vi "GetControlRef.vi"(0 "reference in":refnum<class "MLA.lvclass">, 1 "Control Label":string, 2 "Control Class":string, 5 "error in (no error)":errorcluster) -> (14 "reference out":refnum<class "MLA.lvclass">, 15 "Control":refnum<vi>, 16 "Found?":bool, 19 "error out":errorcluster)   [LabVIEW 2017, in "MLA.lvclass"]
uses:
  MLA.lvclass
  <vilib>/Utility/traverseref.llb/TRef TravTarget.ctl
  <vilib>/Utility/traverseref.llb/VI Scripting - Traverse.lvlib
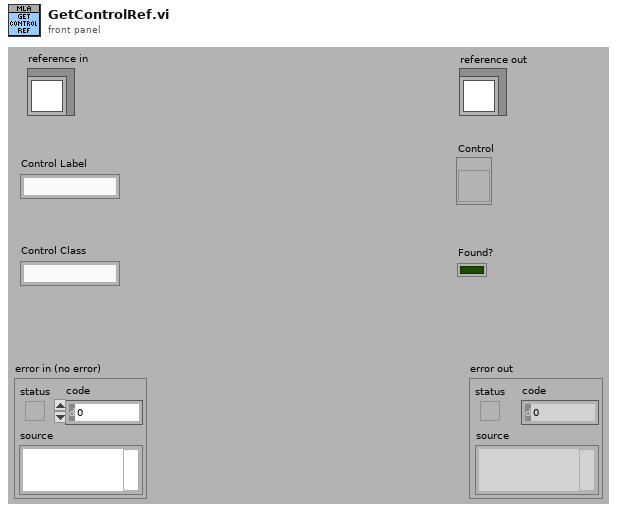
[diagram p1: front panel]
types:
  T1 = typedef "TRef TravTarget.ctl" = enum16{"FP", "BD", "Other"}
  T2 = typedef "MLA.lvclass/ObjectAttributes.ctl" = cluster{"App Name":string, "App Version":string, "Revision History":string, "Log File Path":path, "Config INI File":path, "Config Path":path, "Log Archive Path":path, "Msg Q's":refnum<queue>[], "VI":refnum<vi>, "ErrLog":refnum<class "ErrorLog.lvclass">}
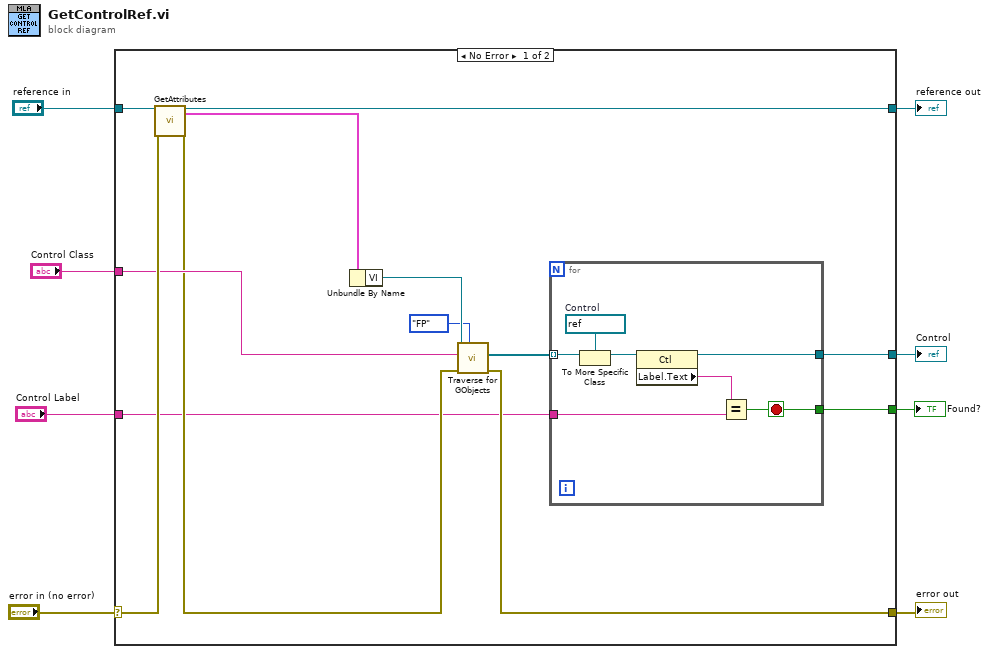
[diagram p0: block diagram]
diagram:
  n1 = case shown="No Error" "error in (no error)" {
    selector: "error in (no error)" -> [w21 w30]
    tunnel: [w14 w30] -> w7
    tunnel: [w18 w29] -> w5
    tunnel: "reference in" -> [w19 w29]
    tunnel: "Control Class" -> [w16 _]
    tunnel: "Control Label" -> [w11 _]
    tunnel: [w10 _] -> w2
    tunnel: [w9 _] -> w1
    frame No Error {
      n2 = call "GetAttributes.vi"("MLA"=w19, "error in (no error)"=w21) -> ("MLA"=w18:refnum<class "MLA.lvclass">, "Data"=w20:T2, "error out"=w15:errorcluster)  [unwired: 14 in, 1 out]
      n3 = Unbundle By Name(w20) -> ("VI"=w17:refnum<vi>)
      n4 = call <vilib>:"Traverse for GObjects.vi"("Traverse Target"=TRef_TravTarget."FP", "error in (no error)"=w15, "Class Name"=w16, "VI Refnum"=w17) -> ("error out"=w14:errorcluster, "References"=w13:refnum<vi>[])  [unwired: 4 in, 2 out]
      n5 = for {
        tunnel: w13 -> [w28] mode=indexing
        tunnel: w11 -> [w24]
        tunnel: [w23] -> w10
        tunnel: [w22] -> w9
        stop <- w22 stop-if-true
        w26 = refnum<vi> refnum  # Control
        n6 = To More Specific Class(target class=w26, reference=w28) -> (specific class reference=w27:refnum<vi>)  [unwired: 1 in, 1 out]
        n7 = property class="Ctl"(reference=w27) -> (reference out=w23:refnum<vi>, "Label.Text"=w25:string)  [unwired: 1 in, 1 out]
        n8 = Equal?(x=w25, y=w24) -> (x = y?=w22:bool)
      }
    }
    frame Error {
    }
  }
  "error out" <- w7
  "reference out" <- w5
  "Control" <- w2
  "Found?" <- w1
